vi "Control de Temperatura.vi"() -> ()   [LabVIEW 2019]
panel:
  in  "RATA DE T° (5°C/Seg)":dbl(knob) scale=0.0..10.0
  in  "Selector":bool
  out "Sensor de Temperatura":i32(slide) scale=0.1..100.0
  # "Incrementar"
  # "Decrementar"
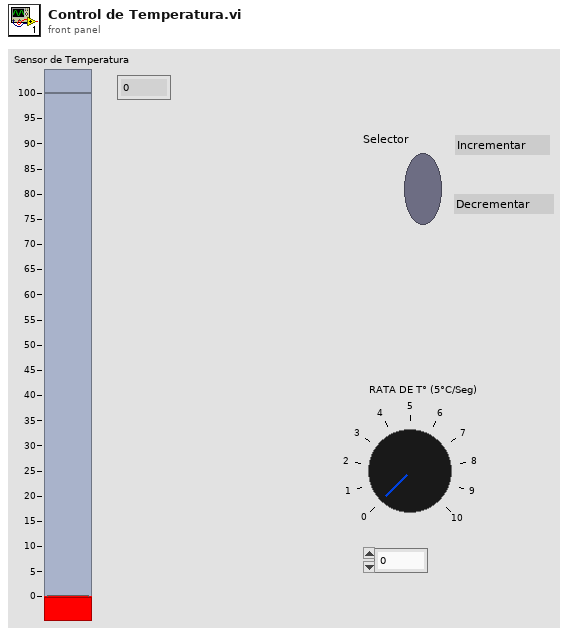
[diagram p1: front panel]
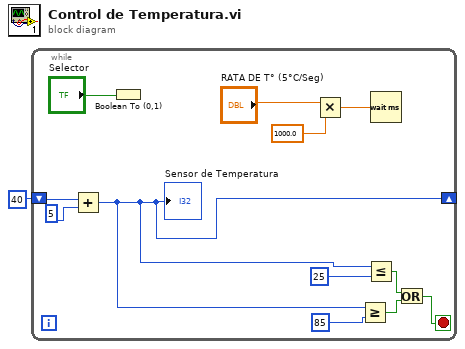
[diagram p0: block diagram]
diagram:
  n1 = while {
    shift-right: [w3] -> _
    shift-left: 40 -> [w5]
    stop <- w13 stop-if-true
    n2 = Add(x=w5, y=5) -> (x+y=w3:i32)
    "Sensor de Temperatura" <- w3
    n3 = Boolean To (0,1)(Boolean="Selector") -> ()  [unwired: 1 out]
    n4 = Multiply(x="RATA DE T° (5°C/Seg)", y=1000.0) -> (x*y=w6:dbl)
    n5 = Greater Or Equal?(x=w3, y=85) -> (x >= y?=w11:bool)
    n6 = Less Or Equal?(x=w3, y=25) -> (x <= y?=w12:bool)
    n7 = Wait (ms)(milliseconds to wait=w6) -> ()  [unwired: 1 out]
    n8 = Or(x=w12, y=w11) -> (x .or. y?=w13:bool)
  }
